vi "Reset All.vi"(7 "index":i32, 8 "error in (no error)":errorcluster, 9 "WL Voltage (V)":dbl, 10 "SL Voltage (V)":dbl, 11 "IVI Refnum in":refnum<k15>) -> (0 "error out":errorcluster, 3 "IVI Refnum out":refnum<k15>)   [LabVIEW 2018]
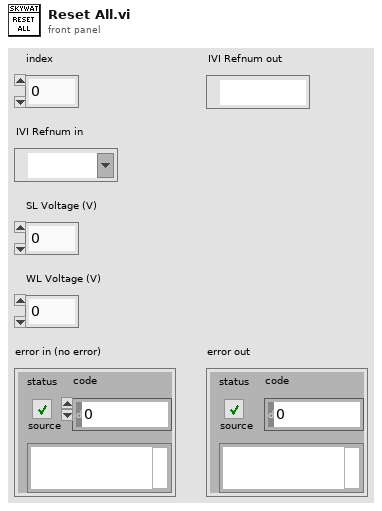
[diagram p1: front panel]
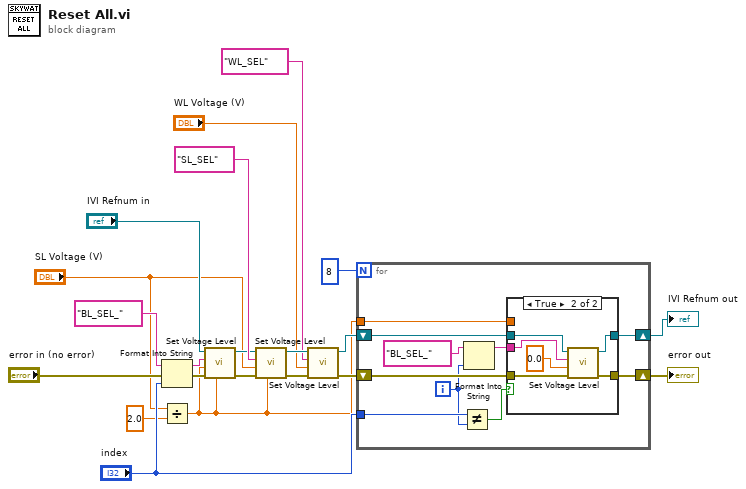
[diagram p0: block diagram]
diagram:
  n1 = Format Into String(initial string="BL_SEL_" ("channel list"), error in="error in (no error)", "index") -> (resulting string=w2:string, error out=w20:errorcluster)  [unwired: 1 in]
  n2 = Divide(x="SL Voltage (V)", y=2.0) -> (x/y=w1:dbl)
  n3 = call "Set Voltage Level.vi"("low level"=w1, "error in (no error)"=w20, "level (V)"=w1, "channel list"=w2, "instrument handle"="IVI Refnum in") -> ("error out"=w16:errorcluster, "instrument handle out"=w17:refnum<k15>)  [unwired: 5 in]
  n4 = call "Set Voltage Level.vi"("low level"=w1, "error in (no error)"=w16, "level (V)"="SL Voltage (V)", "channel list"="SL_SEL", "instrument handle"=w17) -> ("error out"=w3:errorcluster, "instrument handle out"=w8:refnum<k15>)  [unwired: 5 in]
  n5 = call "Set Voltage Level.vi"("error in (no error)"=w3, "level (V)"="WL Voltage (V)", "channel list"="WL_SEL", "instrument handle"=w8) -> ("error out"=w6:errorcluster, "instrument handle out"=w7:refnum<k15>)  [unwired: 6 in]
  n6 = for {
    N: 8 -> [_]
    tunnel: "index" -> [w31]
    shift-right: [w29] -> w12
    shift-left: w7 -> [w30]
    shift-right: [w27] -> w11
    shift-left: w6 -> [w28]
    tunnel: w1 -> [w22]
    i -> [w25]
    n7 = Not Equal?(x=w31, y=w25) -> (x != y?=w26:bool)
    n8 = Format Into String(initial string="BL_SEL_" ("channel list"), w25) -> (resulting string=w23:string)  [unwired: 2 in, 1 out]
    n9 = case shown="True" w26 {
      tunnel: w30 -> [w33 w39]
      tunnel: [w33 w38] -> w29
      tunnel: w28 -> [w32 w37]
      tunnel: [w32 w36] -> w27
      tunnel: w23 -> [_ w35]
      tunnel: w22 -> [_ _]
      frame False {
      }
      frame True {
        n10 = call "Set Voltage Level.vi"("error in (no error)"=w37, "level (V)"=0.0, "channel list"=w35, "instrument handle"=w39) -> ("error out"=w36:errorcluster, "instrument handle out"=w38:refnum<k15>)  [unwired: 6 in]
      }
    }
  }
  "IVI Refnum out" <- w12
  "error out" <- w11
